vi "Untitled 8.vi"() -> ()   [LabVIEW 2013]
panel:
  in  "Сменить предел":bool
  out "range":string
  in  "number":i32
  in  "stop":bool
  out "string":string
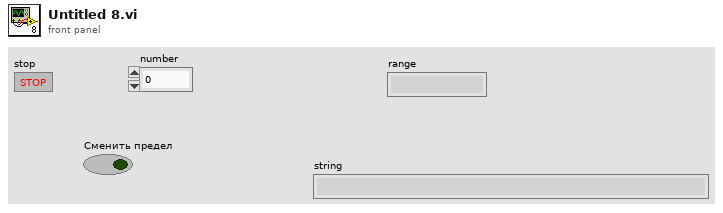
[diagram p1: front panel]
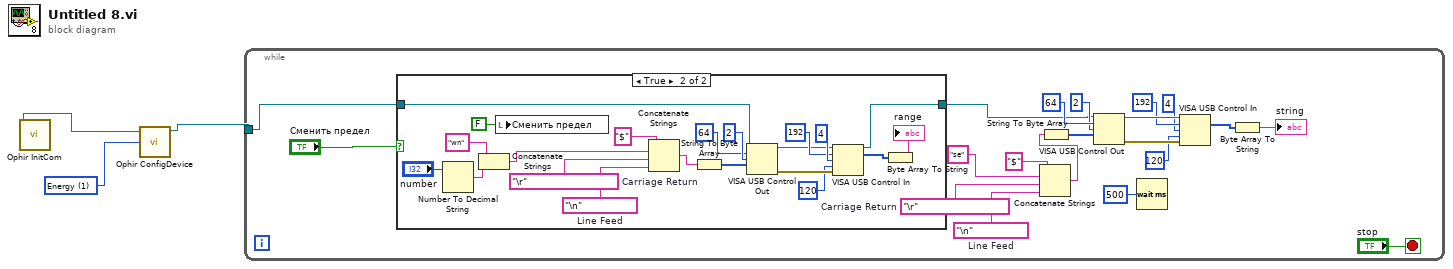
[diagram p0: block diagram]
diagram:
  w2 = u16 1 items=["Power", "Energy", "Frequency"] ("Measure Choice (0:Power)")
  n1 = call "Ophir InitCom.vi"() -> ("Visa Session"=w3:refnum<visa-resource-name>)  [unwired: 6 in, 2 out]
  n2 = call "Ophir ConfigDevice.vi"("Visa Session"=w3, "Measure Choice (0:Power)"=w2) -> ("dup Visa Session"=w1:refnum<visa-resource-name>)  [unwired: 1 in, 3 out]
  n3 = while {
    tunnel: w1 -> [w5]
    stop <- "stop" stop-if-true
    w9 = "\n"  # Line Feed
    w10 = "\r"  # Carriage Return
    n4 = case shown="True" "Сменить предел" {
      tunnel: [w24 w25] -> w6
      tunnel: w5 -> [w24 w26]
      frame False {
      }
      frame True {
        w42 = "\n"  # Line Feed
        w41 = "\r"  # Carriage Return
        n5 = Number To Decimal String(number="number") -> (decimal integer string=w45:string)  [unwired: 1 out]
        n6 = Concatenate Strings("wn", w45) -> (w39:string)
        n7 = local write "Сменить предел"(FALSE ("Сменить предел")) -> ()
        n8 = Concatenate Strings("$", w39, w41, w42) -> (w30:string)
        n9 = String To Byte Array(string=w30) -> (unsigned byte array=w33:u8[])
        n10 = VISA USB Control Out(0:w26, 5:i16 64 ("request type"), 7:i16 2 ("request"), 9:w33) -> (4:w34:refnum<visa-resource-name>, 15:w35:errorcluster)  [unwired: 1 in, 2 out]
        n11 = VISA USB Control In(0:w34, 5:i16 192 ("request type"), 7:i16 4 ("request"), 9:u16 120 ("length (0)"), 11:w35) -> (4:w25:refnum<visa-resource-name>, 6:w38:u8[])  [unwired: 3 out]
        n12 = Byte Array To String(unsigned byte array=w38) -> (string=→"range":string)
      }
    }
    n13 = Concatenate Strings("$", "se" ("string"), w10, w9) -> (w7:string)
    n14 = String To Byte Array(string=w7) -> (unsigned byte array=w21:u8[])
    n15 = VISA USB Control Out(0:w6, 5:i16 64 ("request type"), 7:i16 2 ("request"), 9:w21) -> (4:w20:refnum<visa-resource-name>, 15:w19:errorcluster)  [unwired: 1 in, 2 out]
    n16 = Wait (ms)(milliseconds to wait=u32 500) -> ()  [unwired: 1 out]
    n17 = VISA USB Control In(0:w20, 5:i16 192 ("request type"), 7:i16 4 ("request"), 9:u16 120 ("length (0)"), 11:w19) -> (6:w15:u8[])  [unwired: 4 out]
    n18 = Byte Array To String(unsigned byte array=w15) -> (string=→"string":string)
  }
